vi "rt swap object in dvr.vi"(8 "error in":errorcluster, 10 "module ref in in":refnum<data-value>, 11 "module in":refnum<class "TBM module execution interface.lvclass">) -> (0 "error out":errorcluster, 2 "module ref out":refnum<data-value>, 3 "module out":refnum<class "TBM module execution interface.lvclass">)   [LabVIEW 2013, in "main engine.lvlib"]
uses:
  main engine/main engine.lvlib
  <vilib>/NI/Tag Bus Module Framework/runtime/TBM module execution interface.lvclass
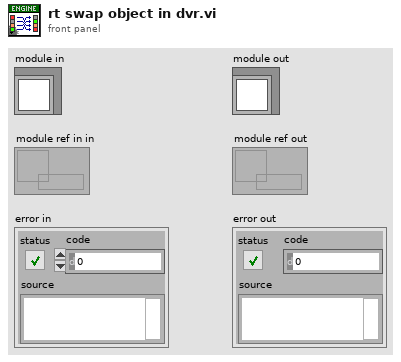
[diagram p1: front panel]
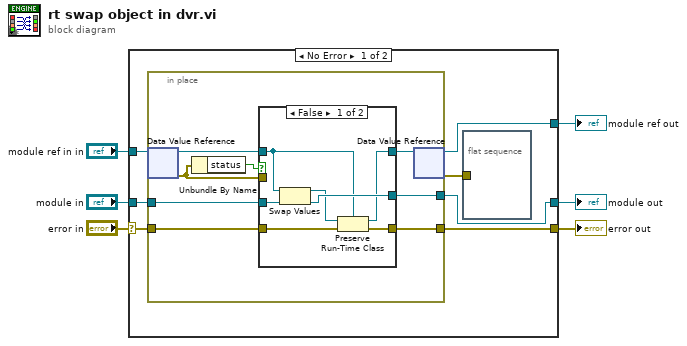
[diagram p0: block diagram]
diagram:
  n1 = case shown="No Error" "error in" {
    selector: "error in" -> [w12 w34]
    tunnel: "module ref in in" -> [w13 w33]
    tunnel: [w11 w34] -> w4
    tunnel: [w10 w33] -> w3
    tunnel: "module in" -> [w8 w32]
    tunnel: [w7 w32] -> w1
    frame No Error {
      n2 = in-place {
        in-place-border: [w21] -> w11
        in-place-border: w12 -> [w20]
        in-place-border: w8 -> [w17]
        in-place-border: [w16] -> w7
        n3 = in-place-dvr #1(w13) -> (w18:refnum<class "TBM module execution interface.lvclass">, w14:errorcluster)
        n4 = Unbundle By Name(w14) -> ("status"=w15:bool)
        n5 = case shown="False" w15 {
          tunnel: [w23 w29] -> w21
          tunnel: w20 -> [w22 _]
          tunnel: [w25 w31] -> w19
          tunnel: w18 -> [w24 w31]
          tunnel: w17 -> [w28 w30]
          tunnel: [w27 w30] -> w16
          tunnel: w14 -> [_ w29]
          frame False {
            n6 = Swap Values(12:w24, 14:w28) -> (1:w26:refnum<class "TBM module execution interface.lvclass">, 3:w27:refnum<class "TBM module execution interface.lvclass">)  [unwired: 1 in]
            n7 = Preserve Run-Time Class(object in=w26, error in=w22, 2:w24) -> (object out=w25:refnum<class "TBM module execution interface.lvclass">, error out=w23:errorcluster)
          }
          frame True {
          }
        }
        n8 = in-place-dvr #1(w19) -> (w10:refnum<data-value>, w9:errorcluster)
      }
      n9 = flat-sequence {
        tunnel: w9 -> [_]
        frame #0 {
        }
      }
    }
    frame Error {
    }
  }
  "error out" <- w4
  "module out" <- w1
  "module ref out" <- w3
